vi "Get Logging Directory.vi"(8 "error in":errorcluster, 11 "logging in":T1=18446744073709551615 format="%.0x") -> (0 "error out":errorcluster, 2 "directory":string, 3 "logging out":T1 format="%.0x")   [LabVIEW 2020, in "AIM MIL-STD-1553 Scripting.lvlib"]
doc: "Returns the directory in which the log file is created."
uses:
  AIM MIL-STD-1553 Scripting.lvlib
  <vilib>/NI VeriStand/Custom Device API/Custom Device Item Ref.ctl
  Constants.vi
  <vilib>/NI VeriStand/Custom Device API/Get Item Property (String).vi
  <vilib>/NI VeriStand/Custom Device API/Custom Device API.lvlib
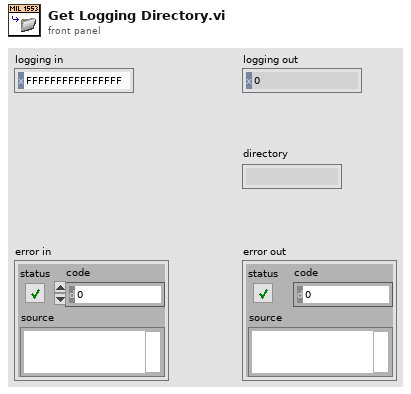
[diagram p1: front panel]
types:
  T1 = typedef "Custom Device API.lvlib/Custom Device Item Ref.ctl" = u64
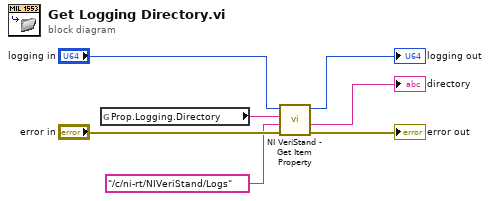
[diagram p0: block diagram]
diagram:
  n1 = global read "Constants.vi" "Prop.Logging.Directory"() -> (w1:string)
  n2 = call-poly <vilib>:"NI VeriStand - Get Item Property.vi"("error in (no error)"="error in", "Default Value"="/c/ni-rt/NIVeriStand/Logs", "Property Name"=w1, "Item Ref in"="logging in") -> ("error out"=→"error out":errorcluster, "Value"=→"directory":string, "Item Ref out"=→"logging out":T1)  [unwired: 4 in, 1 out]
